vi "PicoScope6000Close.vi"(0 "handle":i16) -> ()   [LabVIEW 2020]
doc: "This closes the oscilloscope and should be called before exiting an application."
uses:
  ps6000.dll
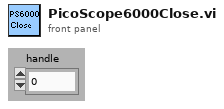
[diagram p1: front panel]
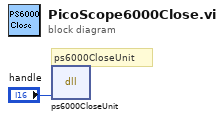
[diagram p0: block diagram]
diagram:
  # "ps6000CloseUnit"
  n1 = dll-call lib="ps6000.dll" fn="ps6000CloseUnit" ("ps3000.dll:_ps3000_open_unit@0")("handle"="handle") -> ()  [unwired: 5 in, 2 out]
